vi "set_display_h2_n2.vi"(0 "Display H2 or N2":bool) -> ()   [LabVIEW 2011]
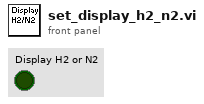
[diagram p1: front panel]
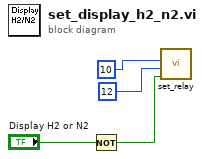
[diagram p0: block diagram]
diagram:
  n1 = Not(x="Display H2 or N2") -> (.not. x?=w4:bool)
  n2 = call "set_relay.vi"("Slot"=10, "Relay"=12, "Relay Status"=w4) -> ()  [unwired: 1 in, 2 out]
